vi "OpenVIs.vi"(8 "error in (no error)":errorcluster, 9 "Title Prefix In":string, 10 "VI Screenshots":T1, 11 "VI Path":path) -> (0 "error out":errorcluster, 2 "VI Screenshots out":T1)   [LabVIEW 2020, in "VIDiffUtilities.lvlib"]
uses:
  VIDiffUtilities.lvlib
  Screenshots/VIScreenshots.ctl
  Screenshots/ScreenshotInfo.ctl
  Screenshots/Screenshot Type.ctl
  FilePaths.ctl
  Screenshots/VIDiffScreenshots.lvlib
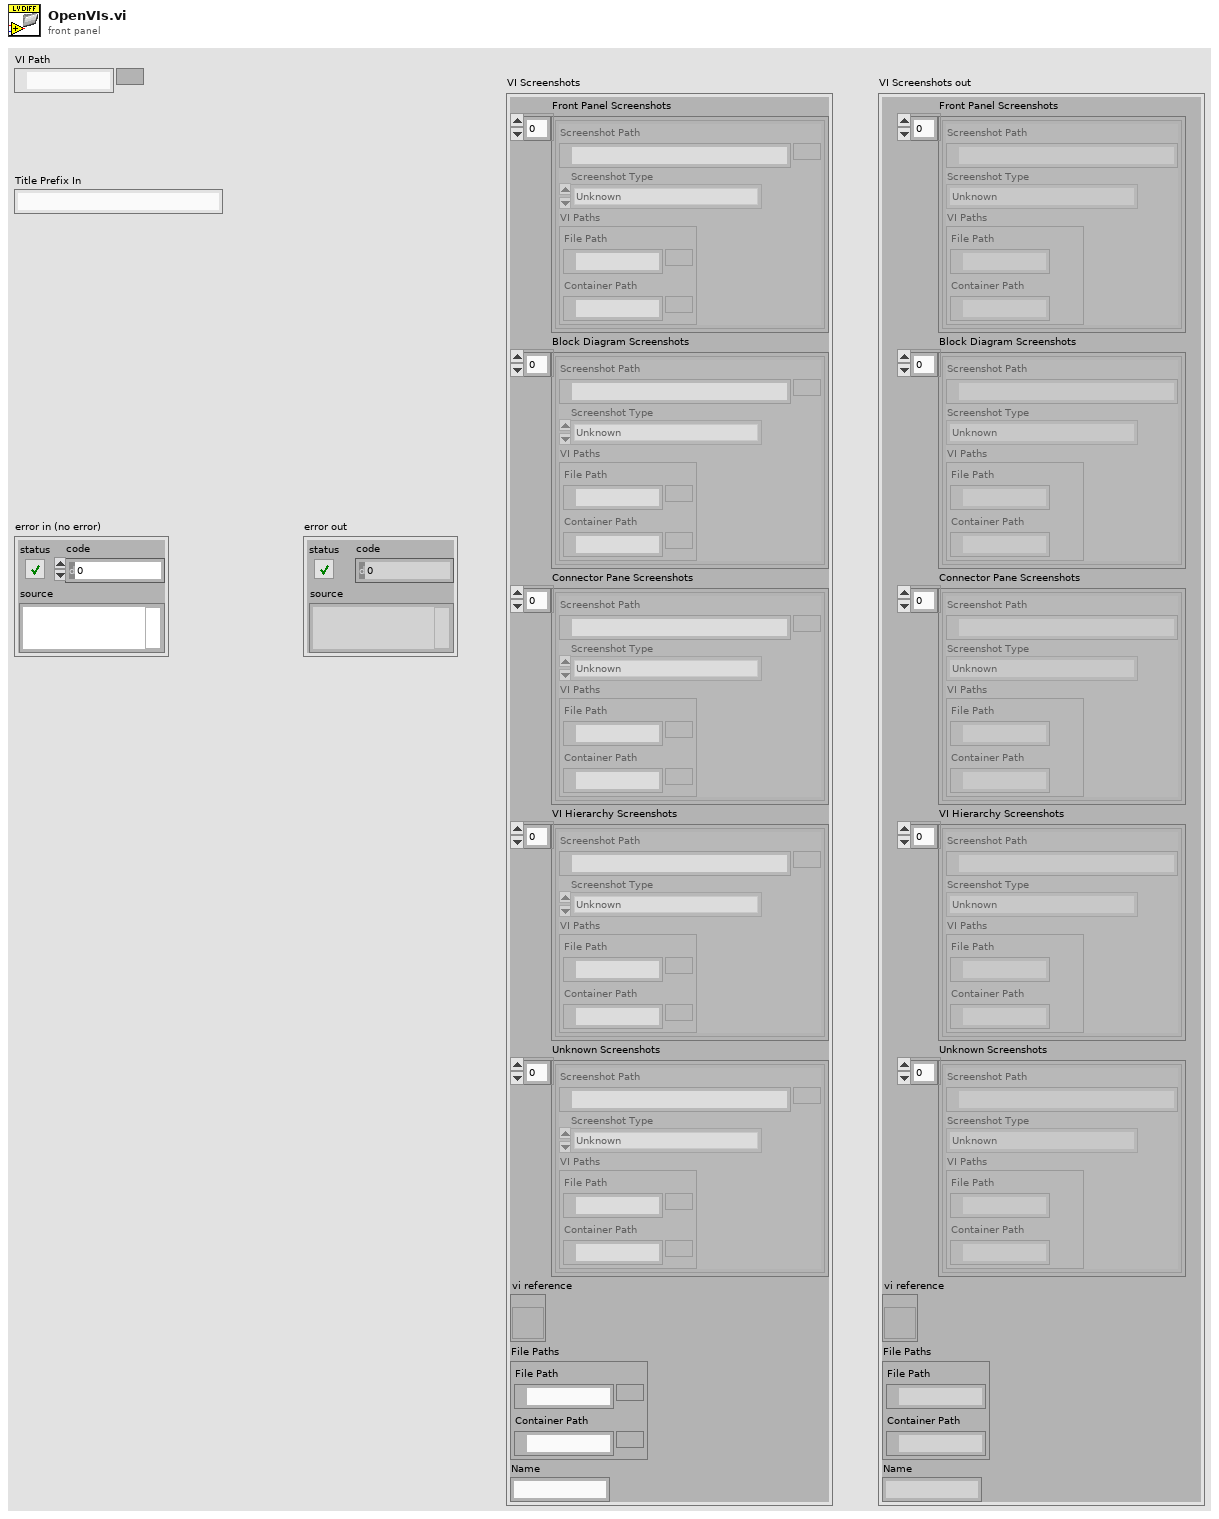
[diagram p1: front panel]
types:
  T1 = typedef "VIDiffScreenshots.lvlib/VIScreenshots.ctl" = cluster{"Front Panel Screenshots":T2[], "Block Diagram Screenshots":T2[], "Connector Pane Screenshots":T2[], "VI Hierarchy Screenshots":T2[], "Unknown Screenshots":T2[], "vi reference":refnum<vi>, "File Paths":cluster{"File Path":path, "Container Path":path}, "Name":string}
  T2 = typedef "VIDiffScreenshots.lvlib/ScreenshotInfo.ctl" = cluster{"Screenshot Path":path, "Screenshot Type":T3, "VI Paths":T4}
  T3 = typedef "VIDiffScreenshots.lvlib/Screenshot Type.ctl" = enum16{"Unknown", "Front Panel", "Connector Pane", "Block Diagram", "VI Hierarchy"}
  T4 = typedef "VIDiffUtilities.lvlib/FilePaths.ctl" = cluster{"File Path":path, "Container Path":path}
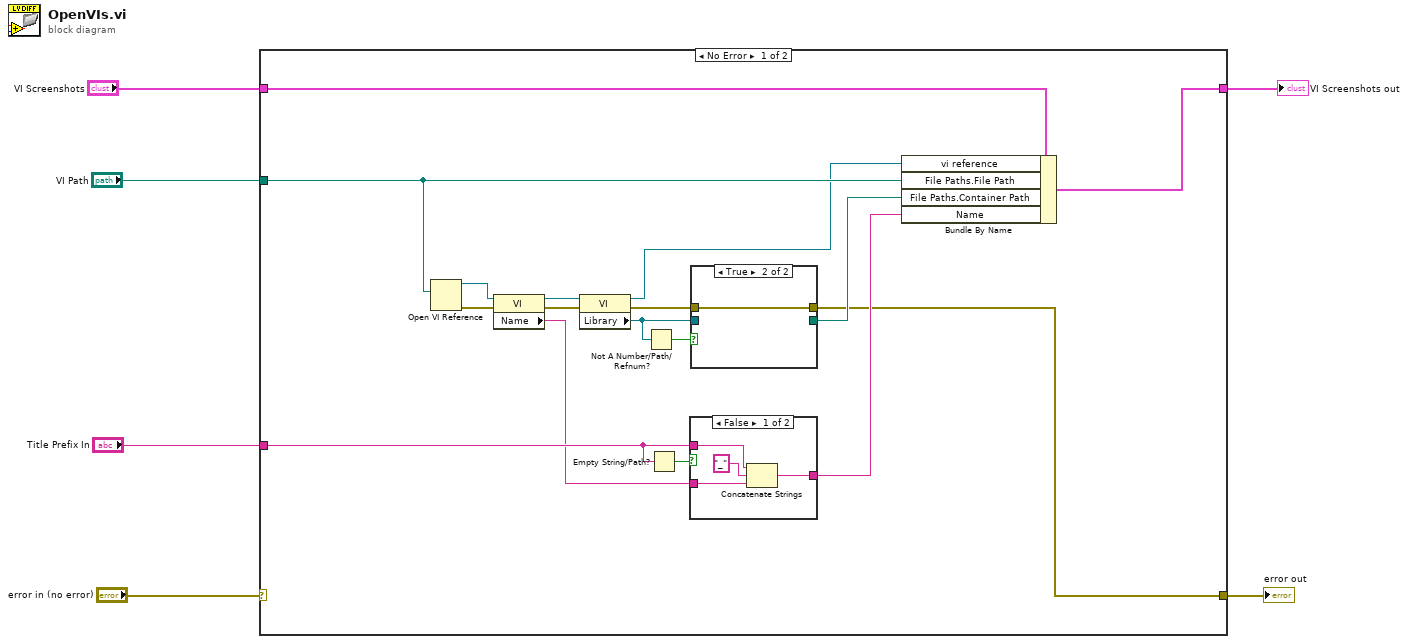
[diagram p0: block diagram]
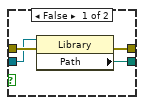
[diagram p3: hidden frame]
diagram:
  n1 = case shown="No Error" "error in (no error)" {
    selector: "error in (no error)" -> [_ w35]
    tunnel: [w7 w35] -> w5
    tunnel: "VI Screenshots" -> [w20 w34]
    tunnel: [w18 w34] -> w3
    tunnel: "VI Path" -> [w17 _]
    tunnel: "Title Prefix In" -> [w10 _]
    frame No Error {
      n2 = Open VI Reference(vi path=w17) -> (vi reference=w16:refnum<vi>, error out=w15:errorcluster)  [unwired: 5 in]
      n3 = property class="VI"(reference=w16, error in=w15) -> (reference out=w13:refnum<vi>, error out=w14:errorcluster, "Name"=w9:string)
      n4 = property class="VI"(reference=w13, error in=w14) -> (reference out=w12:refnum<vi>, error out=w23:errorcluster, "Library"=w21:refnum<vi>)
      n5 = Not A Number/Path/Refnum?(number/path/refnum=w21) -> (NaN/Path/Refnum?=w22:bool)
      n6 = Empty String/Path?(string/path=w10) -> (empty?=w11:bool)
      n7 = case shown="False" w11 {
        tunnel: w9 -> [w27 w28]
        tunnel: [w26 w28] -> w8
        tunnel: w10 -> [w24 _]
        frame False {
          n8 = Concatenate Strings(w24, "_" ("string"), w27) -> (w26:string)
        }
        frame True {
        }
      }
      n9 = case shown="True" w22 {
        tunnel: [w32 _] -> w19
        tunnel: w23 -> [w31 w33]
        tunnel: [w30 w33] -> w7
        tunnel: w21 -> [w29 _]
        frame False {
          n10 = property class="Library"(reference=w29, error in=w31) -> (error out=w30:errorcluster, "Path"=w32:path)  [unwired: 1 out]
        }
        frame True {
        }
      }
      n11 = Bundle By Name(cluster=w20, "vi reference"=w12, "File Paths.File Path"=w17, "File Paths.Container Path"=w19, "Name"=w8) -> (w18:T1)
    }
    frame Error {
    }
  }
  "error out" <- w5
  "VI Screenshots out" <- w3
